vi "Init.vi"(8 "error in (no error)":errorcluster, 11 "Scope PXI Base CFG in":refnum<class "Scope PXI Base CFG.lvclass">) -> (0 "error out":errorcluster, 3 "Scope PXI Base CFG out":refnum<class "Scope PXI Base CFG.lvclass">)   [LabVIEW 2023, in "Scope PXI Base CFG.lvclass"]
uses:
  Scope PXI Base CFG.lvclass
  Scope PXI Base CFG.lvclass/Scope PXI Base CFG.ctl
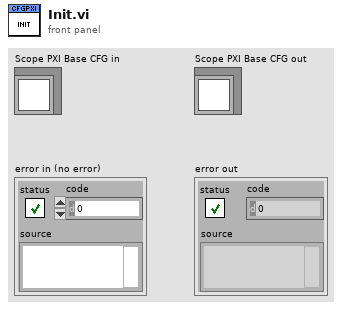
[diagram p1: front panel]
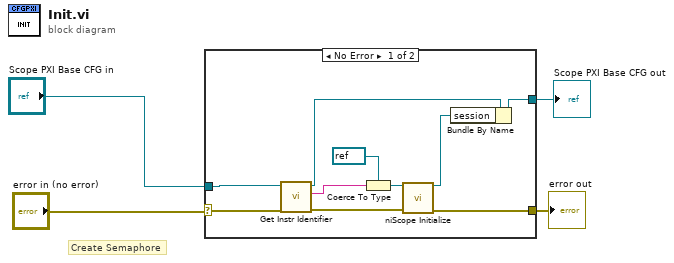
[diagram p0: block diagram]
diagram:
  # "Create Semaphore"
  n1 = case shown="No Error" "error in (no error)" {
    selector: "error in (no error)" -> [w12 w16]
    tunnel: [w14 w16] -> w3
    tunnel: [w13 w15] -> w2
    tunnel: "Scope PXI Base CFG in" -> [w10 w15]
    frame No Error {
      n2 = call-dynamic "Get Instr Identifier.vi"("error in"=w12, "Configuration Base in"=w10) -> ("error out"=w11:errorcluster, "Instr Ident"=w8:string, "Configuration Base out"=w9:refnum<class "Scope PXI Base CFG.lvclass">)  [unwired: 7 in]
      n3 = Coerce To Type(0:w8, 1:refnum<k15> refnum ("resource name")) -> (2:w5:refnum<k15>)
      n4 = call <instrlib>:"niScope Initialize.vi"("resource name"=w5, "error in"=w11) -> ("instrument handle"=w7:refnum<k15>, "error out"=w14:errorcluster)  [unwired: 12 in]
      n5 = Bundle By Name(cluster=w9, "session"=w7) -> (w13:refnum<class "Scope PXI Base CFG.lvclass">)
    }
    frame Error {
    }
  }
  "error out" <- w3
  "Scope PXI Base CFG out" <- w2
